vi "TDMS File Read.vi"(7 "Use input reference (F)":bool, 8 "Error In":errorcluster, 9 "Channel to load":enum16{"Red", "Green", "Both"}(ring)=enum."Both", 10 "tdms file ref":refnum<k34>, 11 "File Path":path) -> (0 "Error Out":errorcluster, 1 "Single channel data":dbl[](array[numeric]), 2 "tdms file out":refnum<k34>, 3 "Data":waveform(dbl)[](array[waveform]))   [LabVIEW 2013]
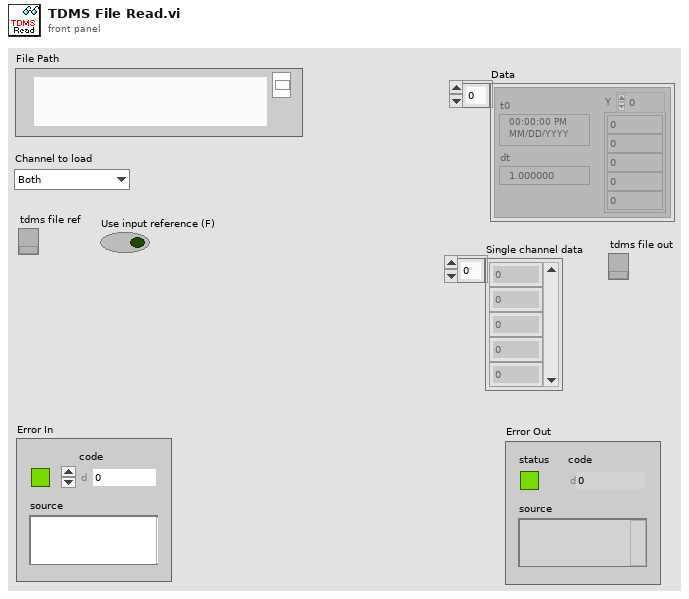
[diagram p1: front panel]
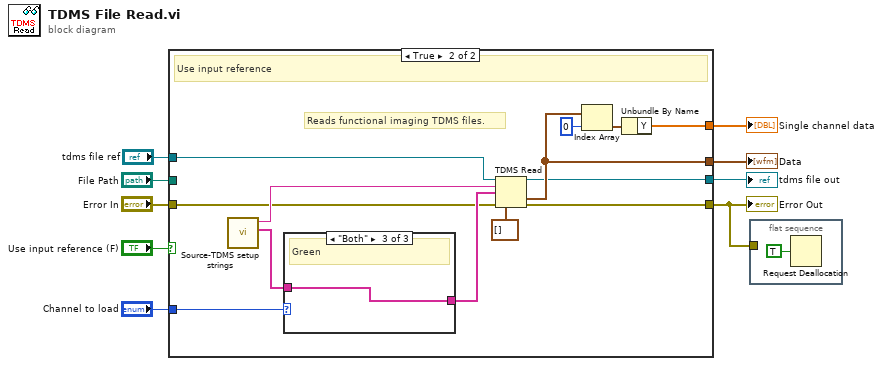
[diagram p0: block diagram]
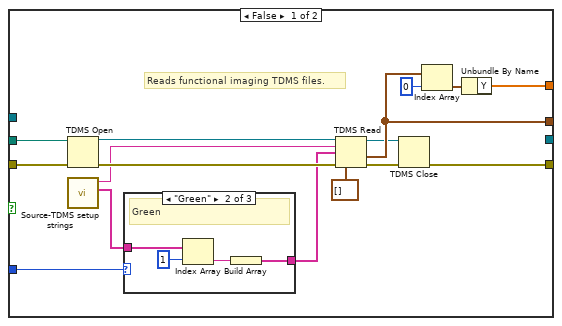
[diagram p2: hidden frame]
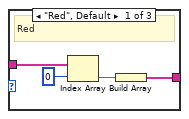
[diagram p3: hidden frame]
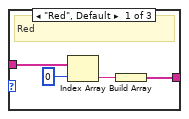
[diagram p5: hidden frame]
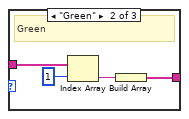
[diagram p6: hidden frame]
diagram:
  n1 = case shown="True" "Use input reference (F)" {
    tunnel: "File Path" -> [w24 _]
    tunnel: "Error In" -> [w20 w35]
    tunnel: [w18 w36] -> w1
    tunnel: "Channel to load" -> [w17 w45]
    tunnel: [w12 w40] -> w6
    tunnel: [w11 w39] -> w5
    tunnel: "tdms file ref" -> [_ w38]
    tunnel: [_ w37] -> w2
    frame False {
      # "Reads functional imaging TDMS files."
      n2 = TDMS Open(8:w20, 11:w24) -> (0:w22:errorcluster, 3:w23:refnum<k34>)  [unwired: 5 in]
      n3 = call "Source-TDMS setup strings.vi"() -> ("Functional imaging TDMS channel names array"=w16:string[], "TDMS group name"=w19:string)  [unwired: 10 in]
      n4 = case shown="\"Green\"" w17 {
        tunnel: [w27 w31 w34] -> w15
        tunnel: w16 -> [w26 w30 w34]
        frame "Red", Default {
          # "Red"
          n5 = Index Array(array=w26, index=0) -> (element=w28:string)
          n6 = Build Array(w28) -> (w27:string[])
        }
        frame "Green" {
          # "Green"
          n7 = Index Array(array=w30, index=1) -> (element=w32:string)
          n8 = Build Array(w32) -> (w31:string[])
        }
        frame "Both" {
          # "Green"
        }
      }
      n9 = TDMS Read(0:w23, 5:w19, 7:w15, 11:w22, 12:waveform(dbl)[] [] ("data type")) -> (4:w10:refnum<k34>, 10:w12:waveform(dbl)[], 15:w21:errorcluster)  [unwired: 3 in, 3 out]
      n10 = TDMS Close(8:w21, 11:w10) -> (0:w18:errorcluster)  [unwired: 1 out]
      n11 = Index Array(array=w12, index=0) -> (element=w14:waveform(dbl))
      n12 = Unbundle By Name ("Get Waveform Components")(w14) -> ("Y"=w11:dbl[])
    }
    frame True {
      # "Reads functional imaging TDMS files."
      # "Use input reference"
      n13 = call "Source-TDMS setup strings.vi"() -> ("Functional imaging TDMS channel names array"=w44:string[], "TDMS group name"=w46:string)  [unwired: 10 in]
      n14 = case shown="\"Both\"" w45 {
        tunnel: [w49 w53 w56] -> w43
        tunnel: w44 -> [w48 w52 w56]
        frame "Red", Default {
          # "Red"
          n15 = Index Array(array=w48, index=0) -> (element=w50:string)
          n16 = Build Array(w50) -> (w49:string[])
        }
        frame "Green" {
          # "Green"
          n17 = Index Array(array=w52, index=1) -> (element=w54:string)
          n18 = Build Array(w54) -> (w53:string[])
        }
        frame "Both" {
          # "Green"
        }
      }
      n19 = TDMS Read(0:w38, 5:w46, 7:w43, 11:w35, 12:waveform(dbl)[] [] ("data type")) -> (4:w37:refnum<k34>, 10:w40:waveform(dbl)[], 15:w36:errorcluster)  [unwired: 3 in, 3 out]
      n20 = Index Array(array=w40, index=0) -> (element=w42:waveform(dbl))
      n21 = Unbundle By Name ("Get Waveform Components")(w42) -> ("Y"=w39:dbl[])
    }
  }
  "Error Out" <- w1
  "Data" <- w6
  "Single channel data" <- w5
  "tdms file out" <- w2
  n22 = flat-sequence {
    tunnel: w1 -> [_]
    frame #0 {
      n23 = Request Deallocation(TRUE ("flag")) -> ()
    }
  }
